vi "Untitled 1.vi"() -> ()   [LabVIEW 2022 SP3]
uses:
  <vilib>/Utility/file.llb/Write Delimited Spreadsheet (DBL).vi
panel:
  in  "file path (dialog if empty)":path
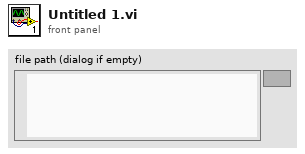
[diagram p1: front panel]
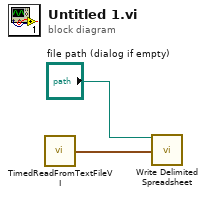
[diagram p0: block diagram]
diagram:
  n1 = call "TimedReadFromTextFileVI.vi"() -> ("Waveform"=w2:waveform(dbl))  [unwired: 12 in, 3 out]
  n2 = call-poly <vilib>:"Write Delimited Spreadsheet.vi"("file path (dialog if empty)"="file path (dialog if empty)", "1D data"=w2) -> ()  [unwired: 12 in, 2 out]
